vi "Lvi Rtd Channel Settings.vi"(0 "TaskRef":i32, 1 "A":dbl, 2 "C":dbl, 3 "DataFilter":u32, 5 "Channel":u32, 7 "RtdType":u32, 9 "NumWireType":u32, 11 "error in (no error)":errorcluster, 12 "B":dbl, 13 "R0":dbl) -> (4 "TaskRef out":i32, 6 "function return":u32(ring), 15 "error out":errorcluster)   [LabVIEW 2022 SP3, in "DtLvLink.lvlib"]
doc: "Calls directly into the entry points of the DLL of the Data Acq SDK to set the bridge configuration."
uses:
  DtLvLink.lvlib
  <userlib>/LV-Link3/DtLvLink_64.dll
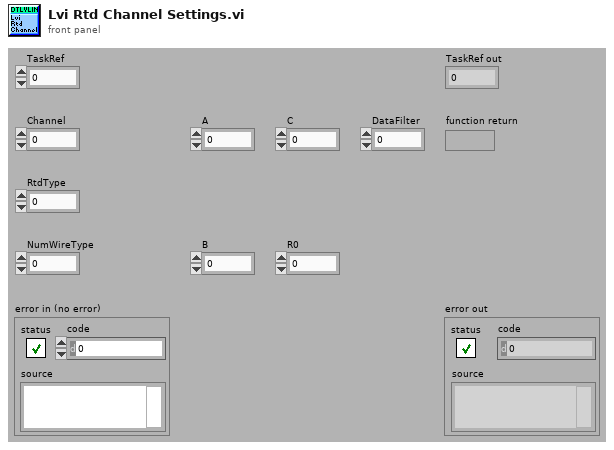
[diagram p1: front panel]
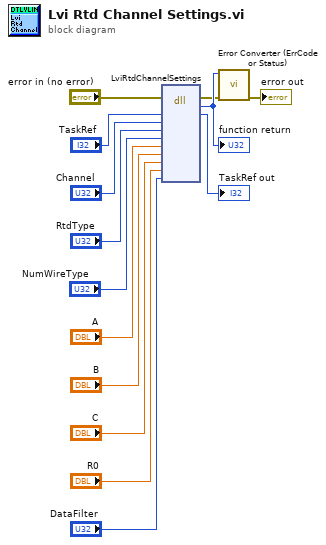
[diagram p0: block diagram]
diagram:
  n1 = dll-call lib="C:/Program Files/National Instruments/LabVIEW 2022/user.lib/LV-Link3/DtLvLink_64.*" fn="LviRtdChannelSettings"(error in="error in (no error)", "TaskRef"="TaskRef", "Channel"="Channel", "RtdType"="RtdType", "NumWireType"="NumWireType", "A"="A", "B"="B", "C"="C", "R0"="R0", "DataFilter"="DataFilter") -> (error out=w2:errorcluster, w14:u32, "TaskRef"=→"TaskRef out":i32)  [unwired: 10 in, 1 out]
  "function return" <- w14
  n2 = call "Error Converter (ErrCode or Status).vi"("error in (no error)"=w2, "error code"=w14) -> ("error out"=→"error out":errorcluster)  [unwired: 9 in]
